vi "Msg.vi"(7 "Actor in":refnum<class "Actor.lvclass">, 11 "Msg Strategy in":refnum<class "Msg Strategy.lvclass">) -> (0 "error out":errorcluster, 5 "Actor out":refnum<class "Actor.lvclass">)   [LabVIEW 2021, in "jettl.lvlib" / "Msg Strategy.lvclass"]
uses:
  Msg Strategy.lvclass
  Actor/Actor.lvclass
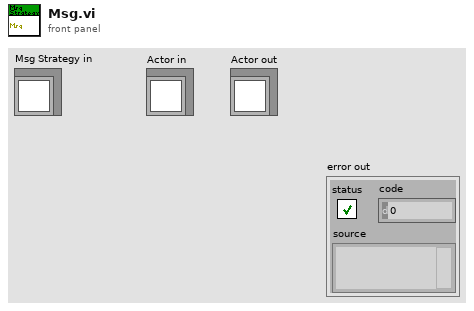
[diagram p1: front panel]
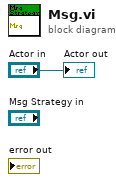
[diagram p0: block diagram]
diagram:
  "Actor out" <- "Actor in"
